vi "拼接Z.vi"(0 "Z高频":cdb[](array[numeric]), 1 "f2":dbl, 5 "Z中频":cdb[](array[numeric]), 7 "f1":dbl, 9 "Z低频":cdb[](array[numeric]), 11 "ff":dbl[](array[numeric]), 12 "f3":dbl) -> (4 "拼接后Z":cluster{"X":dbl, "Y":cdb}[](array[cluster]))   [LabVIEW 2018]
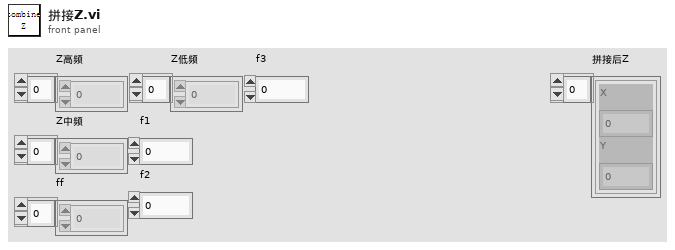
[diagram p1: front panel]
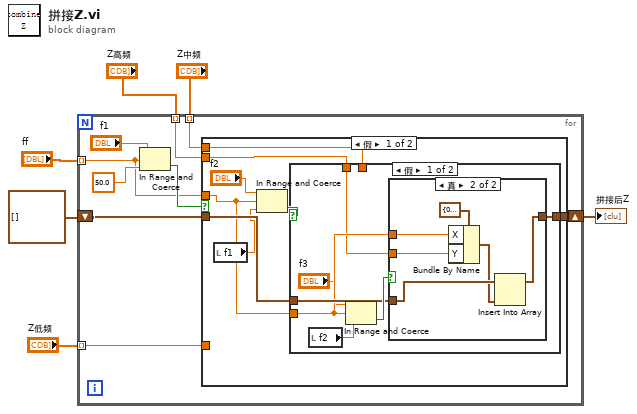
[diagram p0: block diagram]
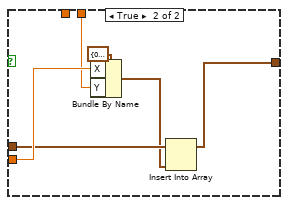
[diagram p3: hidden frame]
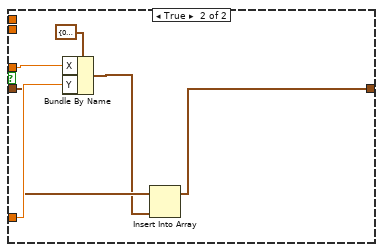
[diagram p4: hidden frame]
diagram:
  n1 = for {
    tunnel: "ff" -> [w12] mode=indexing
    tunnel: "Z低频" -> [w13] mode=indexing
    shift-right: [w11] -> w2
    shift-left: cluster{"X":dbl, "Y":cdb}[] [] ("Z/SI Acoustic Impedance") -> [w10]
    tunnel: "Z中频" -> [w9] mode=indexing
    tunnel: "Z高频" -> [w8] mode=indexing
    n2 = In Range and Coerce(upper limit="f1", x=w12, lower limit=50.0 ("下限")) -> (In Range?=w14:bool)  [unwired: 1 out]
    n3 = case shown="假" w14 {
      tunnel: w13 -> [_ w47]
      tunnel: w12 -> [w21 w48]
      tunnel: [w19 w44] -> w11
      tunnel: w10 -> [w22 w46]
      tunnel: w9 -> [w20 _]
      tunnel: w8 -> [w18 _]
      frame False {
        n4 = local read "f1"() -> (w17:dbl)
        n5 = In Range and Coerce(upper limit="f2", x=w21, lower limit=w17) -> (In Range?=w23:bool)  [unwired: 1 out]
        n6 = case shown="假" w23 {
          tunnel: w22 -> [w29 w40]
          tunnel: w21 -> [w28 w42]
          tunnel: w20 -> [_ w41]
          tunnel: [w26 w38] -> w19
          tunnel: w18 -> [w27 _]
          frame False {
            n7 = local read "f2"() -> (w25:dbl)
            n8 = In Range and Coerce(upper limit="f3", x=w28, lower limit=w25) -> (In Range?=w30:bool)  [unwired: 1 out]
            n9 = case shown="真" w30 {
              tunnel: w29 -> [w31 w36]
              tunnel: w28 -> [_ w34]
              tunnel: w27 -> [_ w33]
              tunnel: [w31 w32] -> w26
              frame False {
              }
              frame True {
                n10 = Bundle By Name(cluster=cluster{"X":dbl, "Y":cdb} {"X"=0.0, "Y"=0.0+0.0i}, "X"=w34, "Y"=w33) -> (w35:cluster{"X":dbl, "Y":cdb})
                n11 = Insert Into Array(array=w36, new element=w35) -> (w32:cluster{"X":dbl, "Y":cdb}[])  [unwired: 1 in]
              }
            }
          }
          frame True {
            n12 = Bundle By Name(cluster=cluster{"X":dbl, "Y":cdb} {"X"=0.0, "Y"=0.0+0.0i}, "X"=w42, "Y"=w41) -> (w39:cluster{"X":dbl, "Y":cdb})
            n13 = Insert Into Array(array=w40, new element=w39) -> (w38:cluster{"X":dbl, "Y":cdb}[])  [unwired: 1 in]
          }
        }
      }
      frame True {
        n14 = Bundle By Name(cluster=cluster{"X":dbl, "Y":cdb} {"X"=0.0, "Y"=0.0+0.0i}, "X"=w48, "Y"=w47) -> (w45:cluster{"X":dbl, "Y":cdb})
        n15 = Insert Into Array(array=w46, new element=w45) -> (w44:cluster{"X":dbl, "Y":cdb}[])  [unwired: 1 in]
      }
    }
  }
  "拼接后Z" <- w2
